vi "biodirection.vi"() -> ()   [LabVIEW 2015]
uses:
  Controls/FPGA_VSYNC State.ctl
  <instrlib>/_niInstr/Basic Elements/v1/FPGA/niInstr Basic Elements v1 FPGA.lvlib
panel:
  in  "Biodirection":bool
  out "波形图表":cluster{i16, "t":i16, i16, i16}(graph)
  in  "SINSYN Trigger":bool
  in  "HSYNC Trigger":bool
  in  "Point":bool
  in  "Start Control":bool=TRUE
  in  "FPGA Stop":bool=TRUE
  in  "Y Step":fxp<+/-,24,16>=1.0
  in  "Line":u32=5
  in  "Y Ramp Step":fxp<+/-,24,16>=1.0
  in  "Back Period":u16
  out "Y Ramp Not State":bool=TRUE
  out "Y Amplitude Full":fxp<+/-,24,16>=3.0 format="%.13g"
  out "VSYNC":bool
  in  "Y Offset":i16
  in  "Y Amplitude":fxp<+,16,0>=0.9999847412109375 format="%.16g"
  out "Y Value":i16=4
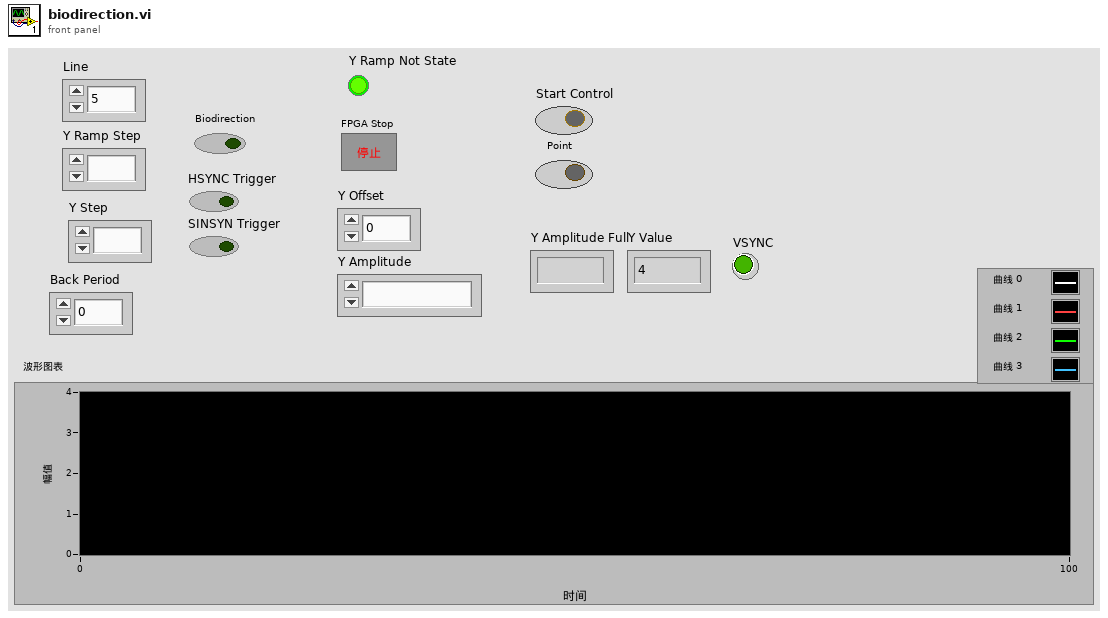
[diagram p1: front panel]
types:
  T1 = typedef "FPGA_VSYNC State.ctl" = enum16{"Initial", "Frame Up", "Wait Frame Up", "Ramp", "Frame Down", "Wait Frame Down"}
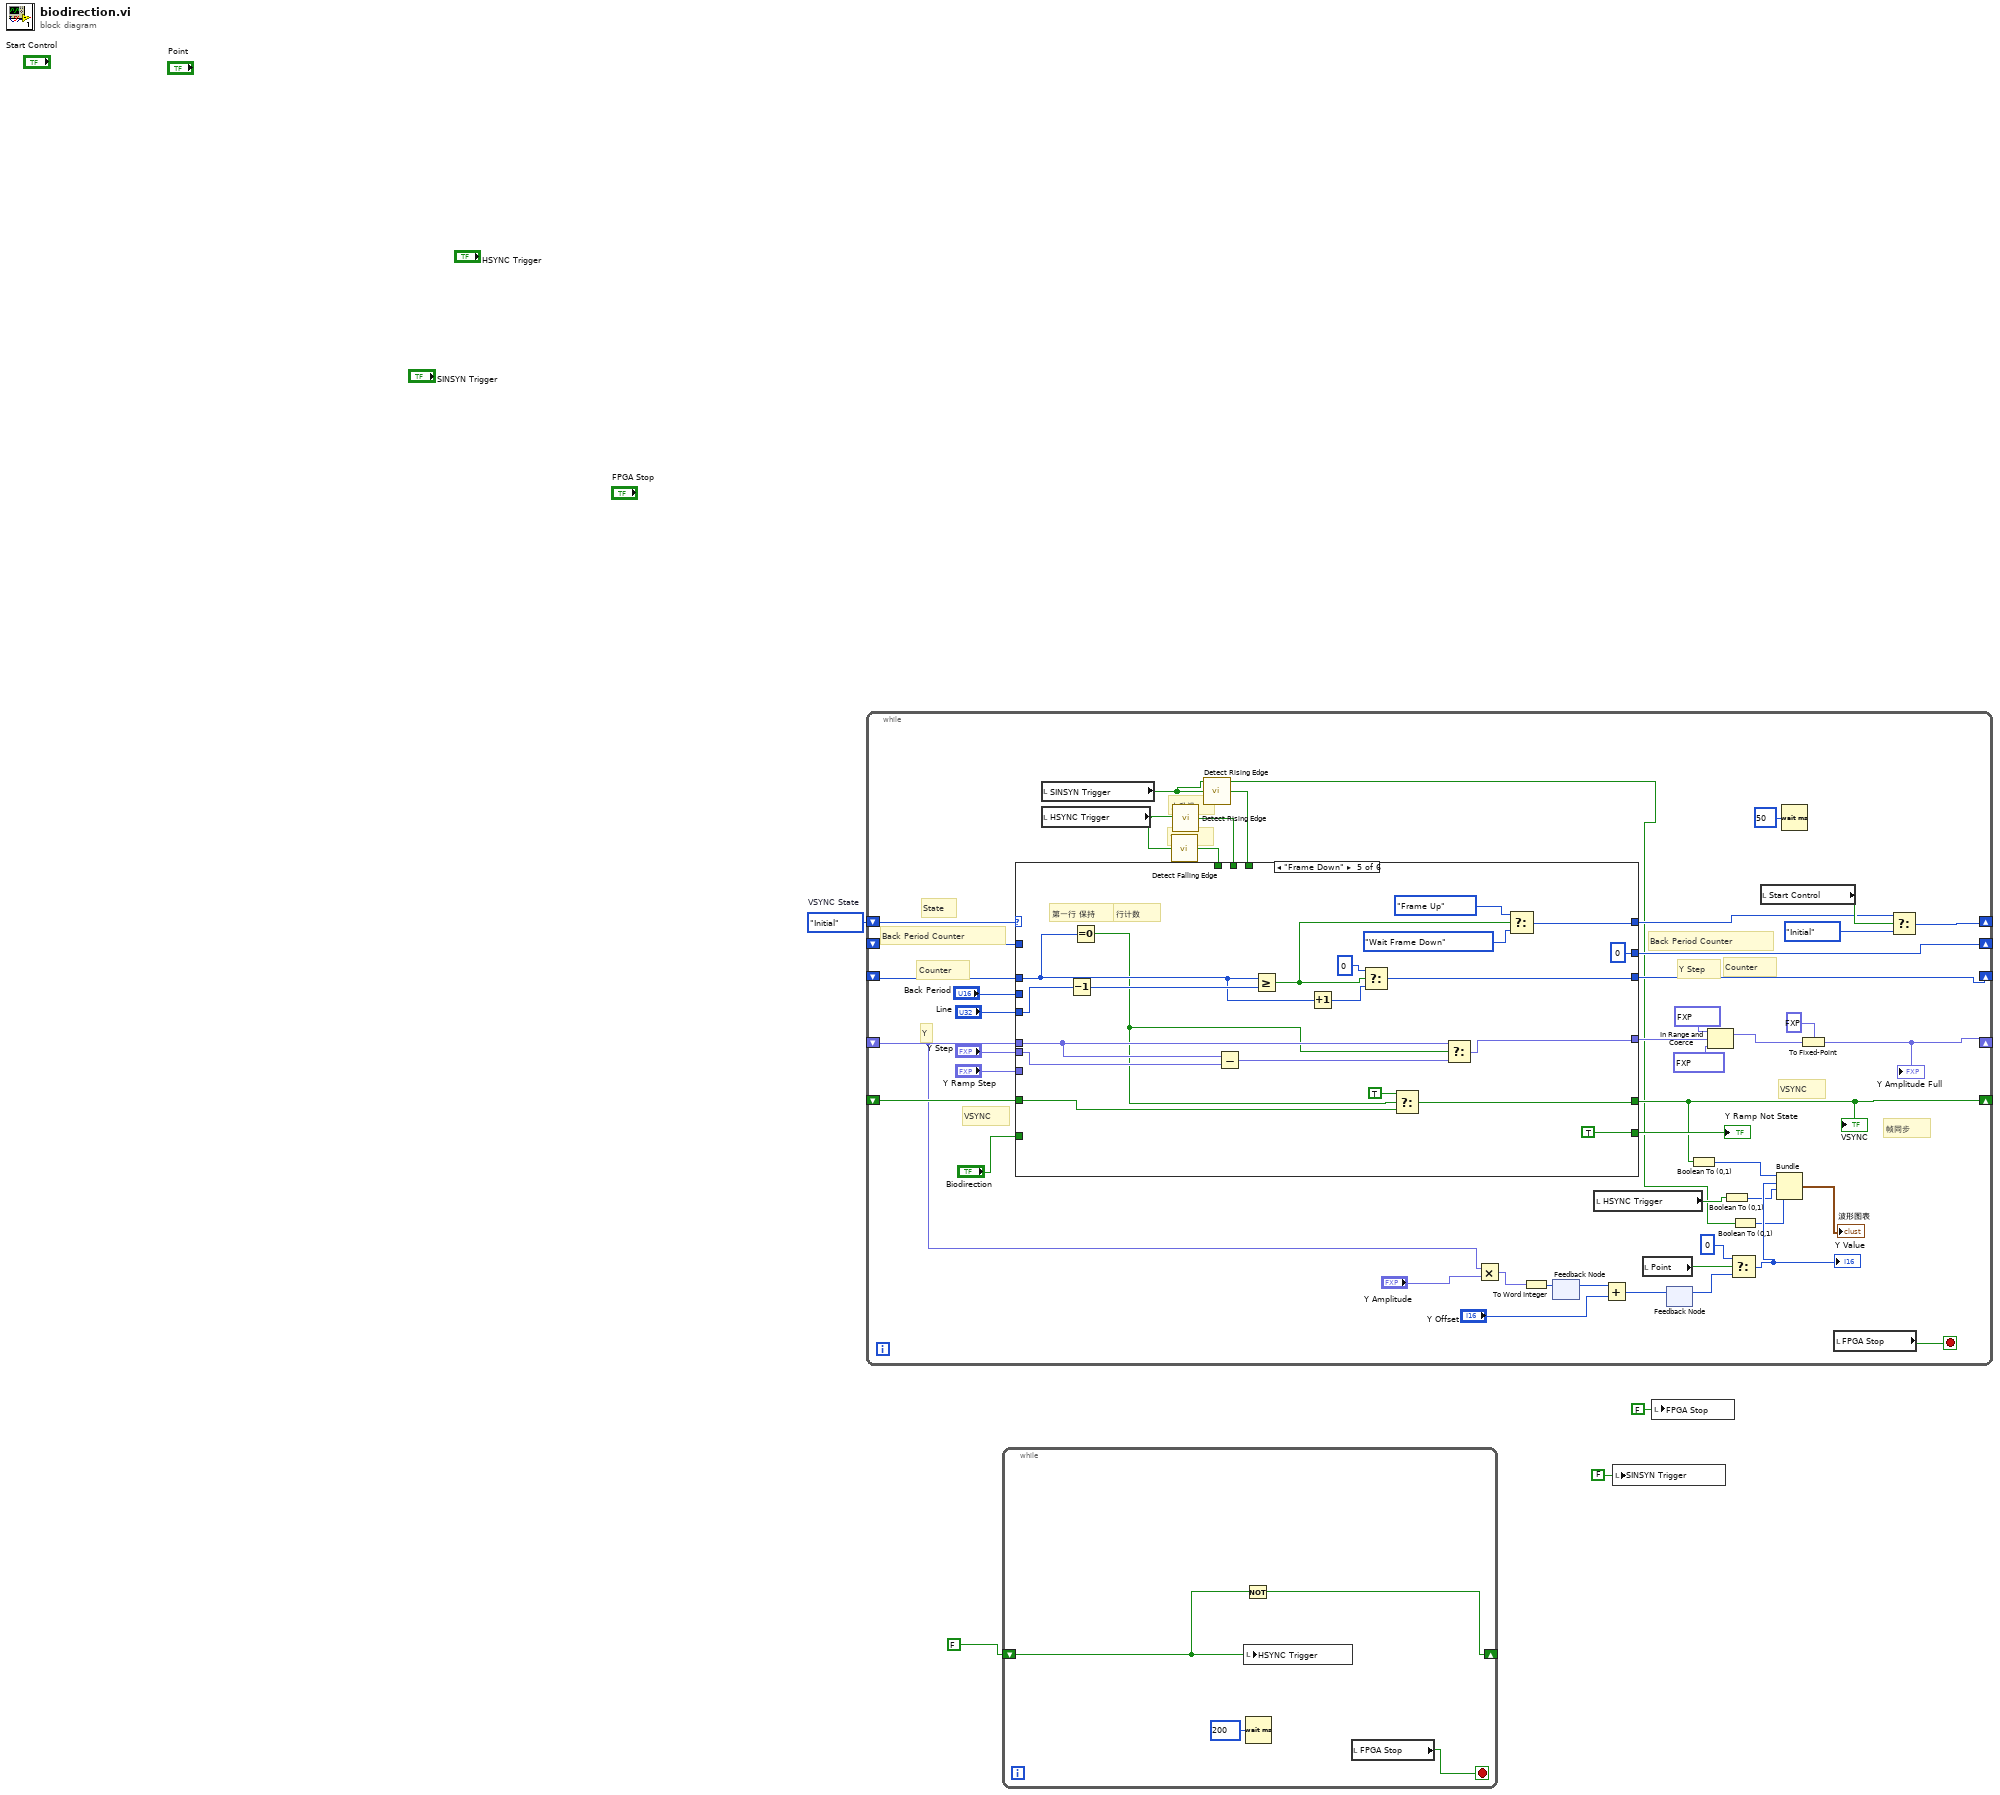
[diagram p0: block diagram]
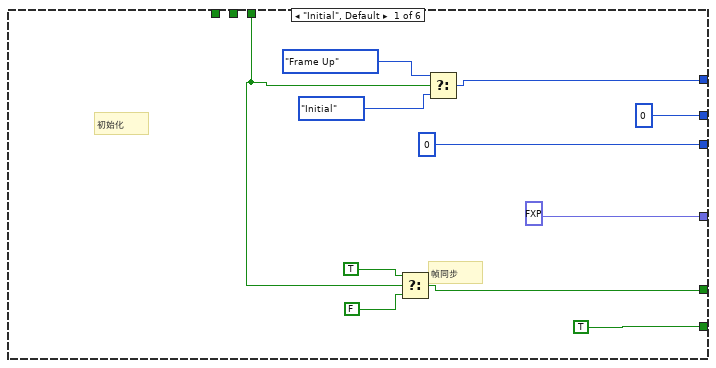
[diagram p2: hidden frame]
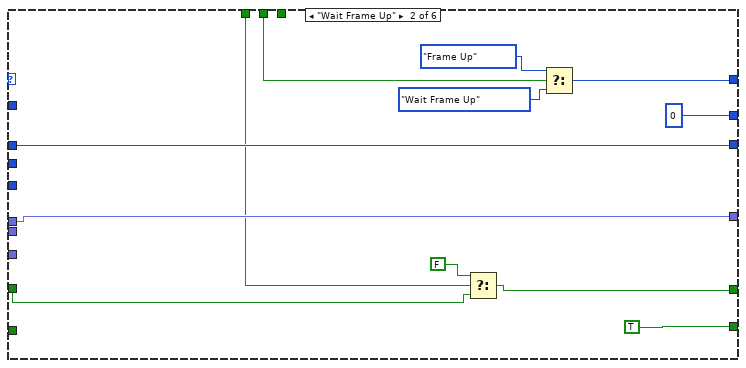
[diagram p3: hidden frame]
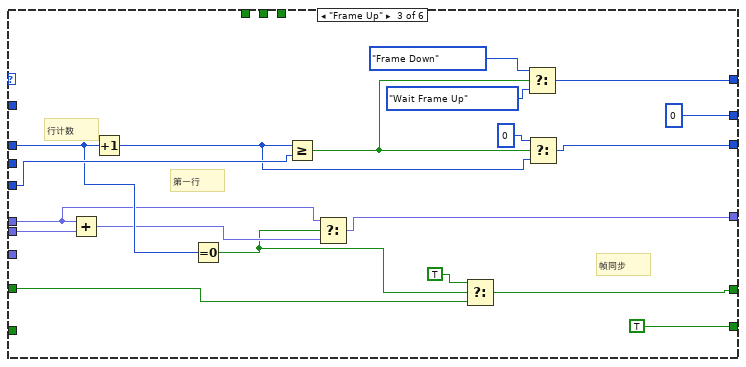
[diagram p4: hidden frame]
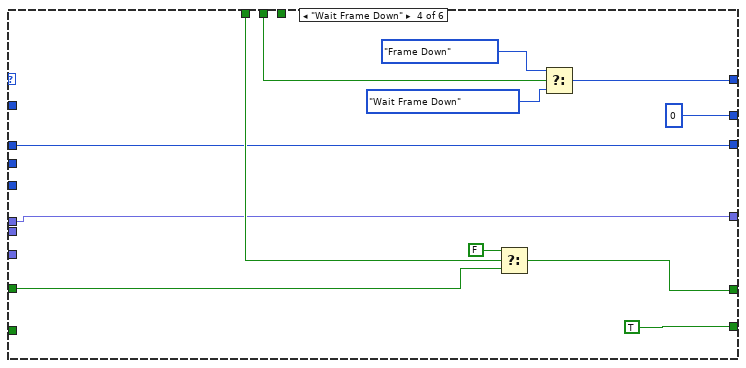
[diagram p5: hidden frame]
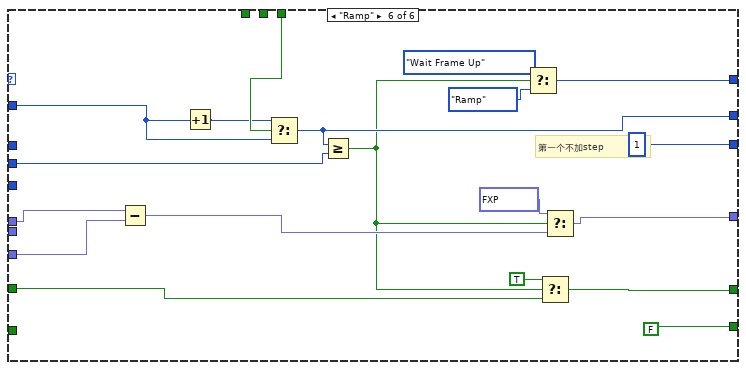
[diagram p6: hidden frame]
diagram:
  w4 = FPGA_VSYNC_State."Initial"  # VSYNC State
  n1 = while {
    shift-right: [w34] -> _
    shift-left: w4 -> [w33]
    shift-right: [w32] -> _
    shift-left: _ -> [w31]
    shift-right: [w30] -> _
    shift-left: _ -> [w29]
    shift-right: [w19] -> _
    shift-left: _ -> [w17]
    shift-right: [w12] -> _
    shift-left: _ -> [w28]
    stop <- w50 stop-if-true
    # "帧同步"
    # "Counter"
    # "Back Period Counter"
    # "Y Step"
    # "下降沿"
    # "上升沿"
    # "Back Period Counter"
    # "VSYNC"
    # "VSYNC"
    # "Counter"
    # "State"
    # "Y"
    n2 = local read "SINSYN Trigger"() -> (w6:bool)
    n3 = local read "HSYNC Trigger"() -> (w27:bool)
    n4 = call <instrlib>:"Detect Falling Edge.vi"("signal"=w27) -> ("edge detected"=w42:bool)  [unwired: 14 in]
    n5 = call <instrlib>:"Detect Rising Edge.vi"("signal"=w27) -> ("edge detected"=w36:bool)  [unwired: 14 in]
    n6 = call <instrlib>:"Detect Rising Edge.vi"("signal"=w6) -> ("edge detected"=w45:bool)  [unwired: 14 in]
    n7 = case shown="\"Frame Down\"" w33 {
      tunnel: [fxp<+/-,24,16> 0.0 ("Y Start") w71 w78 w101 w116 w142] -> w38
      tunnel: [w59 w70 w91 w100 w122 w141] -> w47
      tunnel: w45 -> [w54 _ _ _ _ w134]
      tunnel: [u32 0 w69 w88 w96 w115 u32 1 ("t")] -> w30
      tunnel: w29 -> [_ w69 w81 w96 w107 _]
      tunnel: w17 -> [_ w71 w79 w101 w118 w140]
      tunnel: "Y Step" -> [_ _ w92 _ w109 _]
      tunnel: "Line" -> [_ _ w83 _ w120 _]
      tunnel: [w51 w62 w75 w99 w110 w138] -> w12
      tunnel: w42 -> [_ w63 _ w102 _ _]
      tunnel: w28 -> [_ w64 w76 w98 w106 w137]
      tunnel: "Y Ramp Step" -> [_ _ _ _ _ w143]
      tunnel: w36 -> [_ w68 _ w95 _ _]
      tunnel: w31 -> [_ _ _ _ _ w133]
      tunnel: [u16 0 u16 0 u16 0 u16 0 u16 0 w136] -> w32
      tunnel: "Back Period" -> [_ _ _ _ _ w135]
      tunnel: [TRUE ("Y Ramp State") TRUE ("Y Ramp State") TRUE ("Y Ramp State") TRUE ("Y Ramp State") TRUE ("Y Ramp State") FALSE ("Y Ramp State")] -> w13
      tunnel: "Biodirection" -> [_ _ _ _ _ _]
      frame "Initial", Default {
        # "帧同步"
        # "初始化"
        n8 = Select(t=TRUE, s=w54, f=FALSE ("t")) -> (s? t:f=w51:bool)
        n9 = Select(t=FPGA_VSYNC_State."Frame Up" ("VSYNC State"), s=w54, f=FPGA_VSYNC_State."Initial" ("VSYNC State")) -> (s? t:f=w59:T1)
      }
      frame "Wait Frame Up" {
        n10 = Select(t=FALSE, s=w63, f=w64) -> (s? t:f=w62:bool)
        n11 = Select(t=FPGA_VSYNC_State."Frame Up" ("VSYNC State"), s=w68, f=FPGA_VSYNC_State."Wait Frame Up" ("VSYNC State")) -> (s? t:f=w70:T1)
      }
      frame "Frame Up" {
        # "行计数"
        # "第一行"
        # "帧同步"
        n12 = Add(x=w79, y=w92) -> (x+y=w80:fxp<+/-,25,17>)
        n13 = Increment(x=w81) -> (x+1=w82:u32)
        n14 = Equal To 0?(x=w81) -> (x = 0?=w77:bool)
        n15 = Greater Or Equal?(x=w82, y=w83) -> (x >= y?=w84:bool)
        n16 = Select(t=w79, s=w77, f=w80) -> (s? t:f=w78:fxp<+/-,25,17>)
        n17 = Select(t=TRUE ("Y Ramp State"), s=w77, f=w76) -> (s? t:f=w75:bool)
        n18 = Select(t=FPGA_VSYNC_State."Frame Down" ("VSYNC State"), s=w84, f=FPGA_VSYNC_State."Wait Frame Up" ("VSYNC State")) -> (s? t:f=w91:T1)
        n19 = Select(t=u32 0, s=w84, f=w82) -> (s? t:f=w88:u32)
      }
      frame "Wait Frame Down" {
        n20 = Select(t=FALSE, s=w102, f=w98) -> (s? t:f=w99:bool)
        n21 = Select(t=FPGA_VSYNC_State."Frame Down" ("VSYNC State"), s=w95, f=FPGA_VSYNC_State."Wait Frame Down" ("VSYNC State")) -> (s? t:f=w100:T1)
      }
      frame "Frame Down" {
        # "第一行 保持"
        # "行计数"
        n22 = Decrement(x=w120) -> (x-1=w108:u32)
        n23 = Equal To 0?(x=w107) -> (x = 0?=w105:bool)
        n24 = Subtract(x=w118, y=w109) -> (x-y=w119:fxp<+/-,25,17>)
        n25 = Greater Or Equal?(x=w107, y=w108) -> (x >= y?=w117:bool)
        n26 = Increment(x=w107) -> (x+1=w113:u32)
        n27 = Select(t=u32 0, s=w117, f=w113) -> (s? t:f=w115:u32)
        n28 = Select(t=TRUE, s=w105, f=w106) -> (s? t:f=w110:bool)
        n29 = Select(t=w118, s=w105, f=w119) -> (s? t:f=w116:fxp<+/-,25,17>)
        n30 = Select(t=FPGA_VSYNC_State."Frame Up" ("VSYNC State"), s=w117, f=FPGA_VSYNC_State."Wait Frame Down" ("VSYNC State")) -> (s? t:f=w122:T1)
      }
      frame "Ramp" {
        # "第一个不加step"
        n31 = Subtract(x=w140, y=w143) -> (x-y=w131:fxp<+/-,25,17>)
        n32 = Increment(x=w133) -> (x+1=w126:u16)
        n33 = Select(t=w126, s=w134, f=w133) -> (s? t:f=w136:u16)
        n34 = Greater Or Equal?(x=w136, y=w135) -> (x >= y?=w127:bool)
        n35 = Select(t=FPGA_VSYNC_State."Wait Frame Up" ("VSYNC State"), s=w127, f=FPGA_VSYNC_State."Ramp" ("VSYNC State")) -> (s? t:f=w141:T1)
        n36 = Select(t=TRUE, s=w127, f=w137) -> (s? t:f=w138:bool)
        n37 = Select(t=fxp<+/-,24,16> -32767.0 ("Y Start"), s=w127, f=w131) -> (s? t:f=w142:fxp<+/-,25,17>)
      }
    }
    "Y Ramp Not State" <- w13
    "VSYNC" <- w12
    n38 = Multiply(x=w17, y="Y Amplitude") -> (x*y=w15:fxp<+/-,40,16>)
    n39 = To Word Integer(number=w15) -> (16bit integer=w21:i16)
    n40 = feedback #1() -> (w25:i16)  [unwired: 1 in]
    n41 = feedback-in #1(w21) -> ()
    n42 = local read "HSYNC Trigger"() -> (w8:bool)
    n43 = Add(x=w25, y="Y Offset") -> (x+y=w22:i16)
    n44 = local read "Point"() -> (w24:bool)
    n45 = feedback #2() -> (w26:i16)  [unwired: 1 in]
    n46 = feedback-in #2(w22) -> ()
    n47 = Boolean To (0,1)(Boolean=w12) -> (0, 1=w11:i16)
    n48 = In Range and Coerce(upper limit=fxp<+/-,24,16> 32767.0 ("Y Start"), x=w38, lower limit=fxp<+/-,24,16> -32767.0 ("Y Start")) -> (coerced(x)=w46:fxp<+/-,25,17>)  [unwired: 1 out]
    n49 = Boolean To (0,1)(Boolean=w8) -> (0, 1=w7:i16)
    n50 = Select(t=i16 0, s=w24, f=w26) -> (s? t:f=w10:i16)
    "Y Value" <- w10
    n51 = Boolean To (0,1)(Boolean=w6) -> (0, 1=w5:i16)
    n52 = local read "Start Control"() -> (w49:bool)
    n53 = Bundle(w11, "t"=w10, w7, w5) -> (→"波形图表":cluster{i16, "t":i16, i16, i16})  [unwired: 1 in]
    n54 = Wait (ms)(milliseconds to wait=u32 50 ("等待时间（毫秒）")) -> ()  [unwired: 1 out]
    n55 = To Fixed-Point(fixed-point type=fxp<+/-,24,16> 0.0 ("Y Start"), number=w46) -> (fixed-point=w19:fxp<+/-,24,16>)
    "Y Amplitude Full" <- w19
    n56 = local read "FPGA Stop"() -> (w50:bool)
    n57 = Select(t=w47, s=w49, f=FPGA_VSYNC_State."Initial") -> (s? t:f=w34:T1)
  }
  n58 = while {
    shift-right: [w146] -> _
    shift-left: FALSE ("Y Ramp State") -> [w147]
    stop <- w144 stop-if-true
    n59 = local write "HSYNC Trigger"(w147) -> ()
    n60 = Not(x=w147) -> (.not. x?=w146:bool)
    n61 = Wait (ms)(milliseconds to wait=u32 200 ("等待时间（毫秒）")) -> ()  [unwired: 1 out]
    n62 = local read "FPGA Stop"() -> (w144:bool)
  }
  n63 = local write "SINSYN Trigger"(FALSE ("SINSYN Trigger")) -> ()
  n64 = local write "FPGA Stop"(FALSE ("FPGA Stop")) -> ()
